vi "Ideal Result.vi"(8 "Error in":errorcluster, 11 "DAC in":refnum<class "DAC.lvclass">) -> (0 "Error out":errorcluster, 3 "DAC out":refnum<class "DAC.lvclass">)   [LabVIEW 2020, in "DAC.lvclass"]
uses:
  DAC.lvclass
  Parent/Data Converter/Data Converter.lvclass
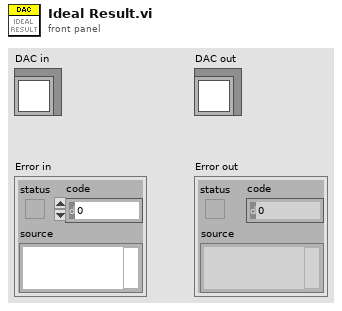
[diagram p1: front panel]
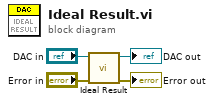
[diagram p0: block diagram]
diagram:
  n1 = call-parent "Ideal Result.vi"("Error in"="Error in", "Device in"="DAC in") -> ("Error out"=→"Error out":errorcluster, "Device out"=→"DAC out":refnum<class "DAC.lvclass">)  [unwired: 8 in]
